vi "Read angles.vi"(8 "error in (no error)":errorcluster, 11 "Position in":refnum<class "Position.lvclass">) -> (0 "error out":errorcluster, 2 "angles":dbl[unit][](array[numeric]), 3 "Position out":refnum<class "Position.lvclass">)   [LabVIEW 2016, in "UnitsAndXML.lvlib" / "Position.lvclass"]
uses:
  <userlib>/Common/UnitsAndXML/SupportFiles/Position/Position.lvclass
  <userlib>/Common/UnitsAndXML/SupportFiles/Position/Position.lvclass/Position.ctl
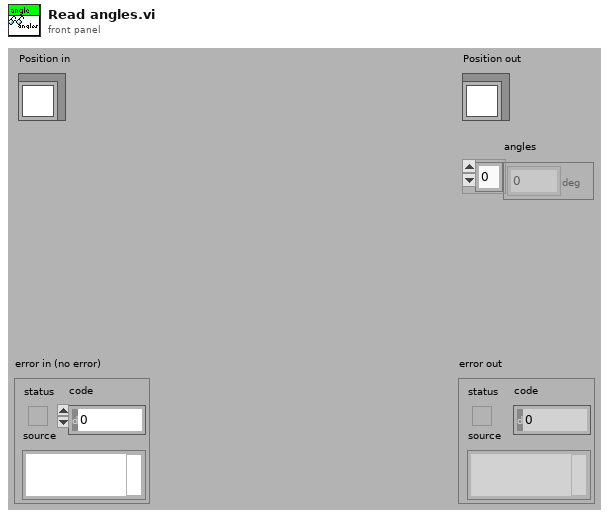
[diagram p1: front panel]
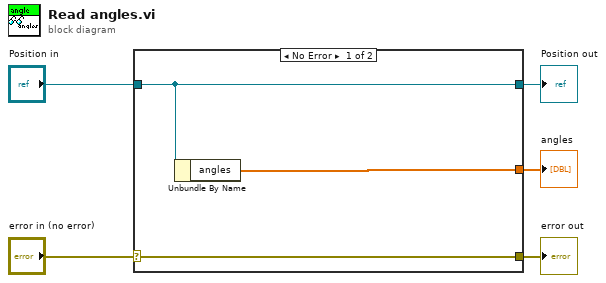
[diagram p0: block diagram]
diagram:
  n1 = case shown="No Error" "error in (no error)" {
    selector: "error in (no error)" -> [w8 w9]
    tunnel: [w8 w9] -> w4
    tunnel: [w7 w10] -> w2
    tunnel: "Position in" -> [w7 w10]
    tunnel: [w6 _] -> w1
    frame No Error {
      n2 = Unbundle By Name(w7) -> ("angles"=w6:dbl[unit][])
    }
    frame Error {
    }
  }
  "error out" <- w4
  "Position out" <- w2
  "angles" <- w1
